vi "读RFID数据.vi"(2 "初始化串口":bool=TRUE caption="写入", 3 "VISA resource name IN":refnum<visa-resource-name>) -> (0 "读取数据":string, 1 "VISA resource name out":refnum<visa-resource-name>)   [LabVIEW 2011]
panel:
  out "read buffer 2":string
  out "error out":errorcluster
  in  "节点地址":i16=2
  out "UID":string
  out "命令码":string
  out "read buffer":string
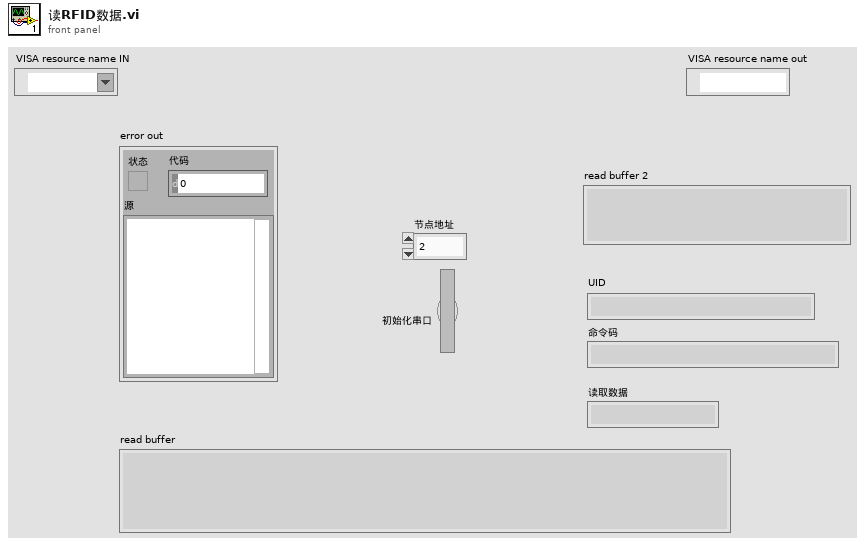
[diagram p1: front panel]
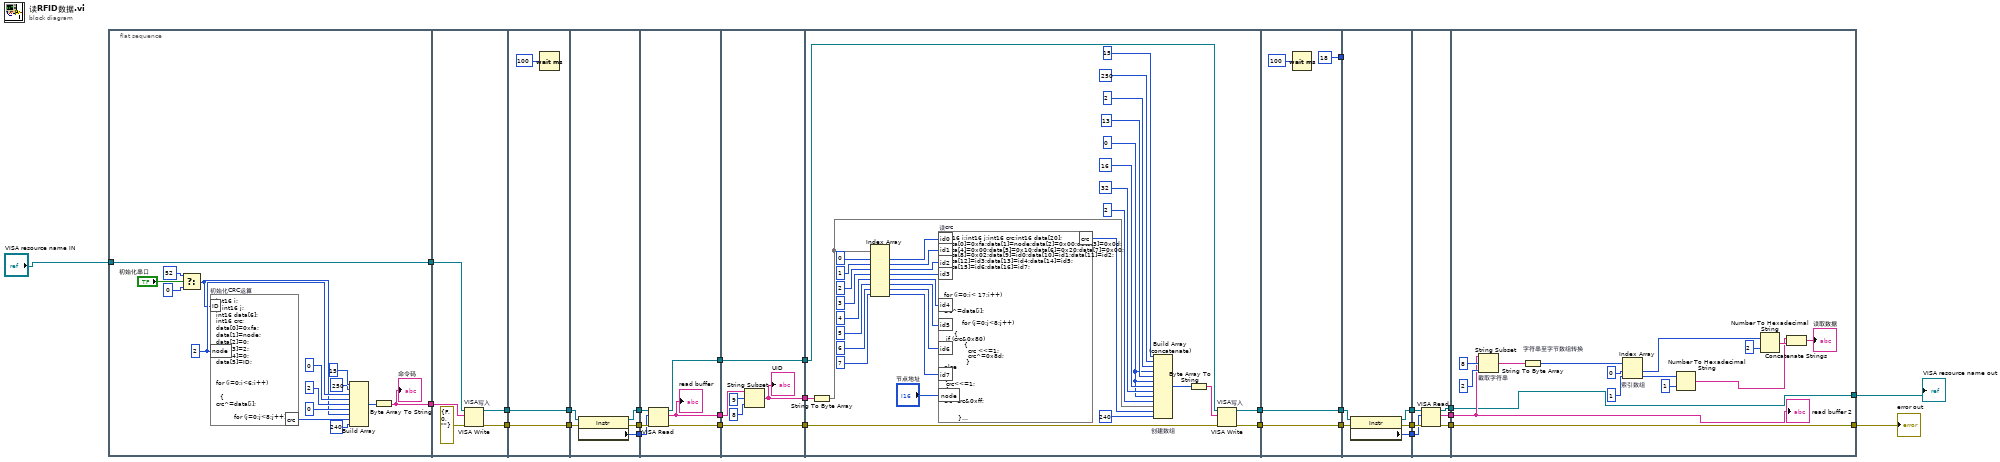
[diagram p0: block diagram]
diagram:
  n1 = flat-sequence {
    tunnel: [w30] -> w29
    tunnel: [w31] -> w28
    tunnel: "VISA resource name IN" -> [w30]
    tunnel: w29 -> [w46]
    tunnel: [w49] -> w27
    tunnel: [w48] -> w26
    tunnel: w28 -> [w47]
    tunnel: w27 -> [w50]
    tunnel: [w50] -> w13
    tunnel: w26 -> [w51]
    tunnel: [w51] -> w11
    tunnel: w13 -> [w56]
    tunnel: [w55] -> w12
    tunnel: w11 -> [w57]
    tunnel: [w53] -> w10
    tunnel: [w54] -> w9
    tunnel: w12 -> [w60]
    tunnel: [w63] -> w25
    tunnel: [w62] -> w24
    tunnel: [w61] -> w23
    tunnel: w10 -> [w58]
    tunnel: w9 -> [w59]
    tunnel: w25 -> [w67]
    tunnel: w24 -> [w65]
    tunnel: [w66] -> w22
    tunnel: [w65] -> w20
    tunnel: [w64] -> w21
    tunnel: w23 -> [w64]
    tunnel: w22 -> [w78]
    tunnel: w21 -> [w75]
    tunnel: w20 -> [w74]
    tunnel: [w71] -> w19
    tunnel: [w70] -> w18
    tunnel: w19 -> [w107]
    tunnel: [w107] -> w8
    tunnel: w18 -> [w106]
    tunnel: [w106] -> w6
    tunnel: [u32 18 ("Serial Settings:Baud Rate")] -> w4
    tunnel: w8 -> [w113]
    tunnel: [w111] -> w7
    tunnel: w6 -> [w112]
    tunnel: [w109] -> w5
    tunnel: w4 -> [_]
    tunnel: [w110] -> w3
    tunnel: w7 -> [w116]
    tunnel: w5 -> [w115]
    tunnel: [w119] -> w17
    tunnel: [w118] -> w16
    tunnel: [w117] -> w15
    tunnel: w3 -> [w114]
    tunnel: w17 -> [w133]
    tunnel: w16 -> [w120]
    tunnel: w15 -> [w122]
    tunnel: [w122] -> w14
    tunnel: [w120] -> w2
    frame #0 {
      w44 = i16 2 ("节点地址")
      n2 = Select(t=52, s="初始化串口", f=0) -> (s? t:f=w33:i32)
      n3 = formula code="int16 i;\n   int16 j;\nint16 data[6];\nint16 crc;\ndata[0]=0xfa;\ndata[1]=node;\ndata[2]=0;\ndata[3]=2;\ndata[4]=0;\ndata[5]=ID;\n\n\nfor (i=0;i<6;i++)\n\n  {\ncrc^=data[i];\n\n         for (j=0;j<8;j++)\n\n     { \n if (crc&0x80)\n          {\n            crc <<=1;\n            crc^=0x8d;\n           }\nelse\n    \n{\n\tcrc<<=1;\n\t}\n\ncrc=crc&0xff;\n\n\n       }\n\n}" "初始化CRC运算"("node"=w44, "ID"=w33) -> ("crc"=w32:i16)
      n4 = Build Array(i16 15 ("数组"), i16 250 ("数组"), w44, i16 0 ("数组"), i16 2 ("数组"), i16 0 ("数组"), w33, w32, i16 240 ("数组")) -> (w43:i32[])
      n5 = Byte Array To String(unsigned byte array=w43) -> (string=w31:string)
      "命令码" <- w31
    }
    frame #1 {
      n6 = VISA Write "VISA写入"(VISA resource name=w46, write buffer=w47, error in (no error)=errorcluster {"status"=FALSE, "code"=0, "source"=""} ("错误输入（无错误）")) -> (VISA resource name out=w49:refnum<visa-resource-name>, error out=w48:errorcluster)  [unwired: 1 out]
    }
    frame #2 {
      n7 = Wait (ms)(milliseconds to wait=u32 100 ("等待时间（毫秒）")) -> ()  [unwired: 1 out]
    }
    frame #3 {
      n8 = property class="Instr"(reference=w56, error in=w57) -> (reference out=w55:refnum<visa-resource-name>, error out=w54:errorcluster, "Serial Settings:Number of Bytes at Serial Port"=w53:u32)
    }
    frame #4 {
      n9 = VISA Read(VISA resource name=w60, byte count=w58, error in (no error)=w59) -> (VISA resource name out=w61:refnum<visa-resource-name>, read buffer=w63:string, error out=w62:errorcluster)  [unwired: 1 out]
      "read buffer" <- w63
    }
    frame #5 {
      n10 = String Subset(string=w67, offset (0)=9 ("偏移量(0)"), length (rest)=8 ("长度（剩余）")) -> (substring=w66:string)
      "UID" <- w66
    }
    frame #6 {
      w98 = i16 0 ("数组")
      n11 = String To Byte Array(string=w78) -> (unsigned byte array=w77:u8[])
      n12 = Index Array(array=w77, index #1=0 ("索引"), index #2=1 ("索引"), index #3=2 ("索引"), index #4=3 ("索引"), index #5=4 ("索引"), index #6=5 ("索引"), index #7=6 ("索引"), index #8=7 ("索引")) -> (element #1=w87:u8, element #2=w88:u8, element #3=w89:u8, element #4=w90:u8, element #5=w91:u8, element #6=w92:u8, element #7=w93:u8, element #8=w94:u8)
      n13 = formula code="int16 i;int16 j;int16 crc;int16 data[20];\ndata[0]=0xfa;data[1]=node;data[2]=0x00;data[3]=0x0d;\ndata[4]=0x00;data[5]=0x10;data[6]=0x20;data[7]=0x00;\ndata[8]=0x02;data[9]=id0;data[10]=id1;data[11]=id2;\ndata[12]=id3;data[13]=id4;data[14]=id5;\ndata[15]=id6;data[16]=id7;\n\n\n\n\nfor (i=0;i< 17;i++)\n\n  {\ncrc^=data[i];\n\n         for (j=0;j<8;j++)\n\n     { \n if (crc&0x80)\n          {\n            crc <<=1;\n            crc^=0x8d;\n           }\nelse\n    \n{\n\tcrc<<=1;\n\t}\n\ncrc=crc&0xff;\n\n\n       }\n\n}" "读crc"("node"="节点地址", "id0"=w87, "id1"=w88, "id2"=w89, "id3"=w90, "id4"=w91, "id5"=w92, "id6"=w93, "id7"=w94) -> ("crc"=w76:i16)
      n14 = Build Array (concatenate) "创建数组"(i16 15 ("数组"), i16 250 ("数组"), i16 2 ("数组"), w98, i16 13 ("数组"), w98, i16 16 ("数组"), i16 32 ("数组"), w98, i16 2 ("数组"), w77, w76, i16 240 ("数组")) -> (w73:i16[])
      n15 = Byte Array To String(unsigned byte array=w73) -> (string=w72:string)
      n16 = VISA Write "VISA写入"(VISA resource name=w75, write buffer=w72, error in (no error)=w74) -> (VISA resource name out=w71:refnum<visa-resource-name>, error out=w70:errorcluster)  [unwired: 1 out]
    }
    frame #7 {
      n17 = Wait (ms)(milliseconds to wait=u32 100 ("等待时间（毫秒）")) -> ()  [unwired: 1 out]
    }
    frame #8 {
      n18 = property class="Instr"(reference=w113, error in=w112) -> (reference out=w111:refnum<visa-resource-name>, error out=w109:errorcluster, "Serial Settings:Number of Bytes at Serial Port"=w110:u32)
    }
    frame #9 {
      n19 = VISA Read(VISA resource name=w116, byte count=w114, error in (no error)=w115) -> (VISA resource name out=w118:refnum<visa-resource-name>, read buffer=w119:string, error out=w117:errorcluster)  [unwired: 1 out]
    }
    frame #10 {
      n20 = String Subset "截取字符串"(string=w133, offset (0)=8 ("偏移量(0)"), length (rest)=2 ("长度（剩余）")) -> (substring=w130:string)
      n21 = String To Byte Array "字符串至字节数组转换"(string=w130) -> (unsigned byte array=w128:u8[])
      n22 = Index Array "索引数组"(array=w128, index #1=0 ("索引"), index #2=1 ("索引")) -> (element #1=w132:u8, element #2=w125:u8)
      n23 = Number To Hexadecimal String ("数值至十六进制字符串转换")(1:i16 1 ("宽度(-)"), 2:w125) -> (0:w121:string)
      n24 = Number To Hexadecimal String ("数值至十六进制字符串转换")(1:i16 2 ("宽度(-)"), 2:w132) -> (0:w123:string)
      n25 = Concatenate Strings(w121, w123) -> (→"读取数据":string)
      "read buffer 2" <- w133
    }
  }
  "error out" <- w14
  "VISA resource name out" <- w2
